vi "PH_BeamlineController.set i Attr.vi"() -> (0 "PH_BeamlineController.i attribute":T1 {"Status Tags"."Status" items=["no info", "off/false/out", "on/true/in", "Failure", "Alarm", "Status 1", "Status 2", "Status 3"]})   [LabVIEW 2014, in "PH_BeamlineController.lvlib"]
uses:
  PH_BeamlineController.lvlib
  PH_BeamlineController.i attribute.ctl
  PH_BeamlineController.Source Attributes.ctl
  PH_BeamlineController.Sources.ctl
  PH_BeamlineController.PA DP Target Attributes.ctl
  PH_BeamlineController.PA DP Targets.ctl
  PH_BeamlineController.Targets.ctl
  PH_Basics/PH_StatusHandler/PH_StatusHandler.Status.ctl
  PH_BeamlineController.special GUI Refs.ctl
  PH_Beamline/PH_Beamline.Black Box Instances.ctl
  PH_Beamline/PH_Beamline.6P Switch Instances.ctl
  PH_Beamline/PH_Beamline.Switch Instances.ctl
  PH_Basics/PH_StatusHandler/PH_StatusHandler.lvlib
  PH_Beamline/PH_Beamline.lvlib
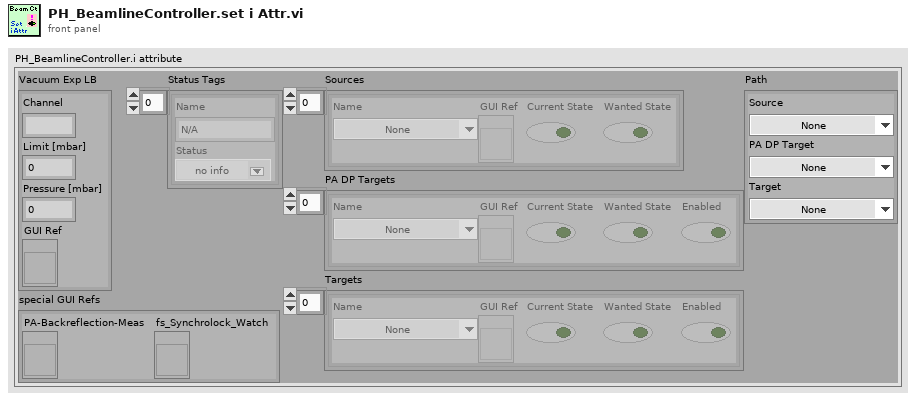
[diagram p1: front panel]
types:
  T1 = typedef "PH_BeamlineController.lvlib/PH_BeamlineController.i attribute.ctl" = cluster{"Vacuum Exp LB":cluster{"Channel":string, "Limit [mbar]":dbl, "Pressure [mbar]":dbl, "GUI Ref":refnum<vi>}, "Sources":T2[], "PA DP Targets":T4[], "Path":cluster{"Source":T3, "PA DP Target":T5, "Target":T6}, "Targets":cluster{"Name":T6, "GUI Ref":refnum<vi>, "Current State":bool, "Wanted State":bool, "Enabled":bool}[], "Status Tags":cluster{"Name":string, "Status":T7}[], "special GUI Refs":T8}
  T2 = typedef "PH_BeamlineController.lvlib/PH_BeamlineController.Source Attributes.ctl" = cluster{"Name":T3, "GUI Ref":refnum<vi>, "Current State":bool, "Wanted State":bool}
  T3 = typedef "PH_BeamlineController.lvlib/PH_BeamlineController.Sources.ctl" = enum16{"None", "YLF", "fs-Frontend", "ns-Frontend", "YLF and ns-Frontend", "fs- and ns-Frontend"}
  T4 = typedef "PH_BeamlineController.lvlib/PH_BeamlineController.PA DP Target Attributes.ctl" = cluster{"Name":T5, "GUI Ref":refnum<vi>, "Current State":bool, "Wanted State":bool, "Enabled":bool}
  T5 = typedef "PH_BeamlineController.lvlib/PH_BeamlineController.PA DP Targets.ctl" = enum16{"None", "Dump PA Delayed Beam", "Dump PA Undelayed Beam", "Dumps PA Delayed and Undelayed Beam"}
  T6 = typedef "PH_BeamlineController.lvlib/PH_BeamlineController.Targets.ctl" = enum16{"None", "PreAmp", "Dump Exp Laserlab", "Exp Laserlab", "Calorimeter", "Dump Exp Laserbay", "Exp Laserbay", "Dump Exp Z6", "Exp Z6"}
  T7 = typedef "PH_StatusHandler.lvlib/PH_StatusHandler.Status.ctl" = i16
  T8 = typedef "PH_BeamlineController.lvlib/PH_BeamlineController.special GUI Refs.ctl" = cluster{"PA-Backreflection-Meas":refnum<vi>, "fs_Synchrolock_Watch":refnum<vi>}
  T9 = typedef "PH_Beamline.lvlib/PH_Beamline.Switch Instances.ctl" = string
  T10 = typedef "PH_Beamline.lvlib/PH_Beamline.6P Switch Instances.ctl" = string
  T11 = typedef "PH_Beamline.lvlib/PH_Beamline.Black Box Instances.ctl" = string
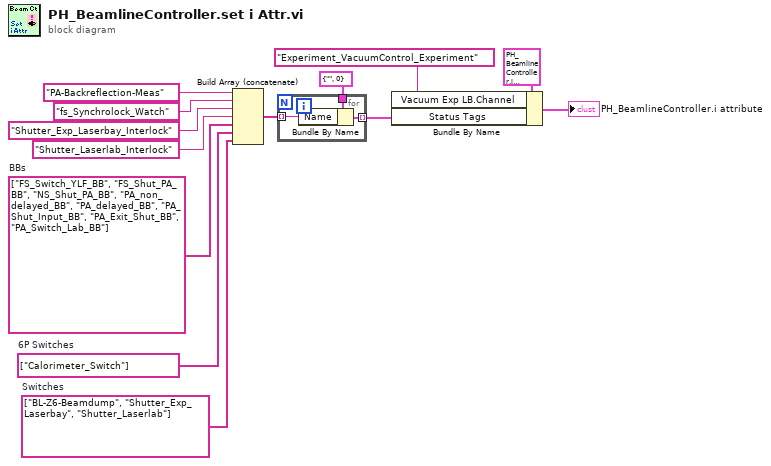
[diagram p0: block diagram]
diagram:
  w13 = T9[] ["BL-Z6-Beamdump", "Shutter_Exp_Laserbay", "Shutter_Laserlab"]  # Switches
  w12 = T10[] ["Calorimeter_Switch"]  # 6P Switches
  w10 = T11[] ["FS_Switch_YLF_BB", "FS_Shut_PA_BB", "NS_Shut_PA_BB", "PA_non_delayed_BB", "PA_delayed_BB", "PA_Shut_Input_BB", "PA_Exit_Shut_BB", "PA_Switch_Lab_BB"]  # BBs
  n1 = Build Array (concatenate)("PA-Backreflection-Meas" ("Instance PA Backreflection"), "fs_Synchrolock_Watch" ("Synchrolock.Instance"), "Shutter_Exp_Laserbay_Interlock" ("Instance PA Backreflection"), "Shutter_Laserlab_Interlock" ("Instance PA Backreflection"), w10, w12, w13) -> (w11:T9[])
  n2 = for {
    tunnel: [w16] -> w4 mode=indexing
    tunnel: cluster{"Name":string, "Status":T7} {"Name"="", "Status"=0} ("Tag") -> [w15]
    tunnel: w11 -> [w14] mode=indexing
    n3 = Bundle By Name(cluster=w15, "Name"=w14) -> (w16:cluster{"Name":string, "Status":T7})
  }
  n4 = Bundle By Name(cluster=T1 {"Vacuum Exp LB"={"Channel"="N/A", "Limit [mbar]"=0.0, "Pressure [mbar]"=0.0, "GUI Ref"=refnum}, "Sources"=[], "PA DP Targets"=[], "Path"={"Source"=enum."None", "PA DP Target"=enum."None", "Target"=enum."None"}, "Targets"=[], "Status Tags"=[], "special GUI Refs"={"PA-Backreflection-Meas"=refnum, "fs_Synchrolock_Watch"=refnum}} ("CLASS.i attribute"), "Vacuum Exp LB.Channel"="Experiment_VacuumControl_Experiment" ("Vacuum Exp LB.Instance"), "Status Tags"=w4) -> (→"PH_BeamlineController.i attribute":T1)
